vi "IRAdressData.vi"() -> ()   [LabVIEW 2023]
panel:
  out "Data":bool[](array[boolean])
  in  "Data":u8 format="%x"
  out "Adresse":bool[](array[boolean])
  in  "Adresse":u8
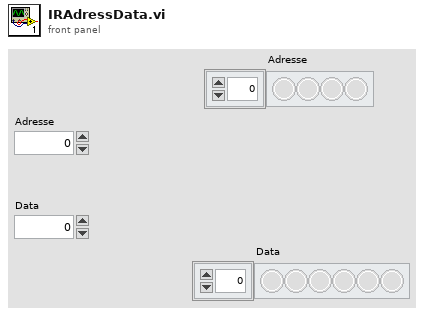
[diagram p1: front panel]
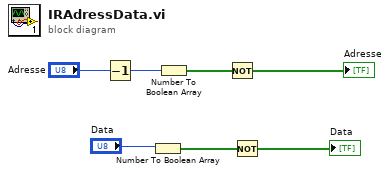
[diagram p0: block diagram]
diagram:
  n1 = Decrement(x="Adresse") -> (x-1=w1:u8)
  n2 = Number To Boolean Array(number="Data") -> (Boolean array=w4:bool[])
  n3 = Number To Boolean Array(number=w1) -> (Boolean array=w6:bool[])
  n4 = Not(x=w6) -> (.not. x?=→"Adresse":bool[])
  n5 = Not(x=w4) -> (.not. x?=→"Data":bool[])
